vi "mainActivity_刷新界面控件.vi"(10 "控件索引2":T1, 11 "控件索引1":T2) -> (0 "错误输出":errorcluster)   [LabVIEW 2014]
uses:
  glb/glb_static.vi
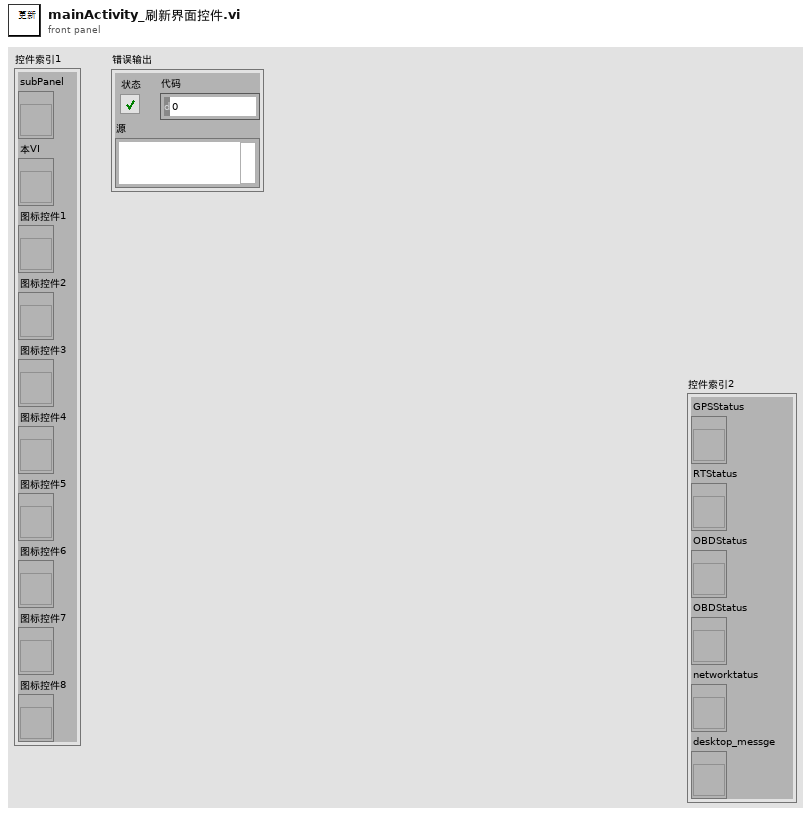
[diagram p1: front panel]
types:
  T1 = cluster{"GPSStatus":refnum<vi>, "RTStatus":refnum<vi>, "OBDStatus":refnum<vi>, "OBDStatus":refnum<vi>, "networktatus":refnum<vi>, "desktop_messge":refnum<vi>}
  T2 = cluster{"subPanel":refnum<vi>, "本VI":refnum<vi>, "图标控件1":refnum<vi>, "图标控件2":refnum<vi>, "图标控件3":refnum<vi>, "图标控件4":refnum<vi>, "图标控件5":refnum<vi>, "图标控件6":refnum<vi>, "图标控件7":refnum<vi>, "图标控件8":refnum<vi>}
  T3 = cluster{"标题":string, "相对路径":string, "类型":enum16{"服务", "活动"}, "专属队列名称":string}[]
  T4 = enum32{"Bad", "Idle", "Run top level", "Running"}
  T5 = cluster{"侧边栏数据":cluster{"来源":string, "名称":string}[], "界面刷间隔率":dbl}
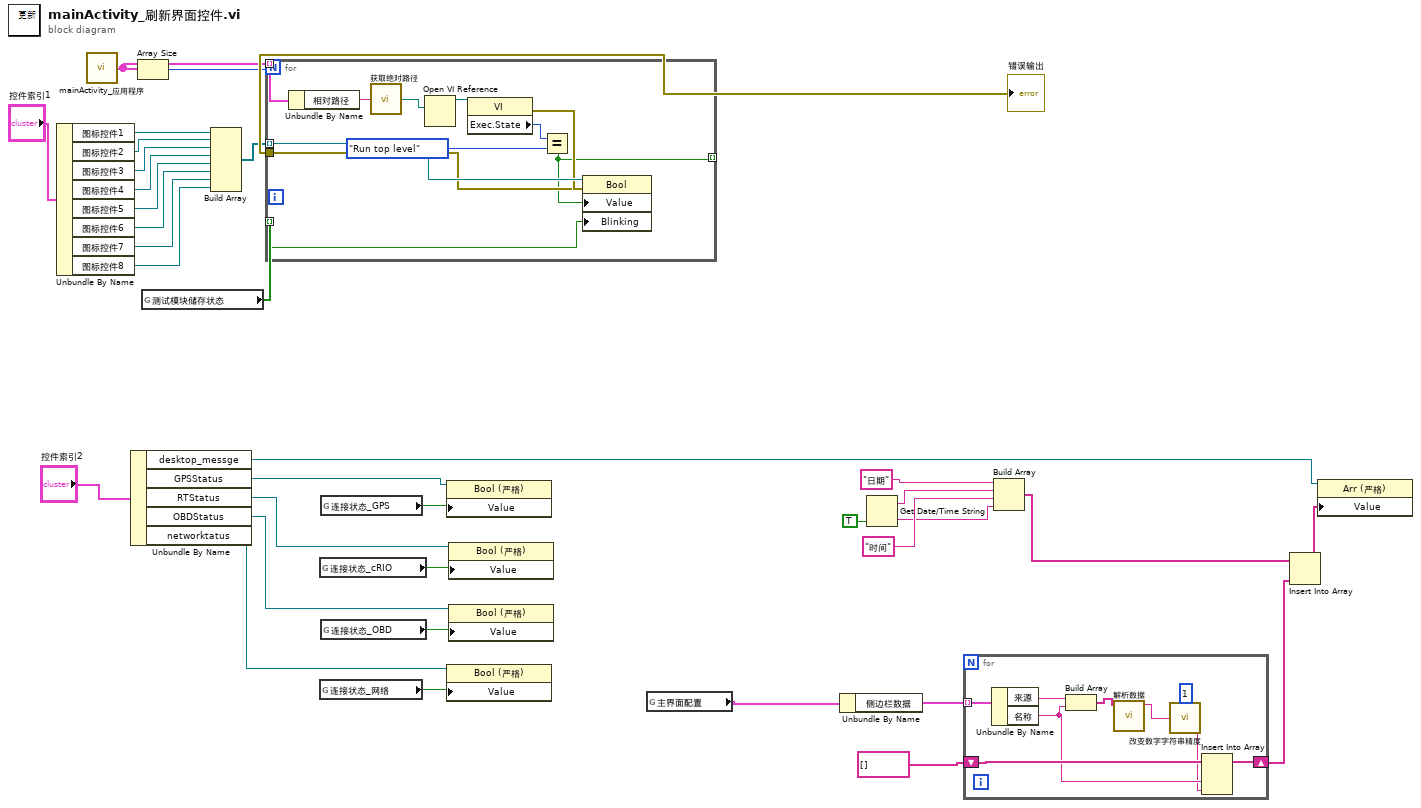
[diagram p0: block diagram]
diagram:
  n1 = Unbundle By Name("控件索引1") -> ("图标控件1"=w23:refnum<vi>, "图标控件2"=w24:refnum<vi>, "图标控件3"=w25:refnum<vi>, "图标控件4"=w26:refnum<vi>, "图标控件5"=w28:refnum<vi>, "图标控件6"=w29:refnum<vi>, "图标控件7"=w30:refnum<vi>, "图标控件8"=w31:refnum<vi>)
  n2 = call "mainActivity_应用程序.vi"() -> ("应用"=w33:T3)
  n3 = Unbundle By Name("控件索引2") -> ("desktop_messge"=w3:refnum<vi>, "GPSStatus"=w20:refnum<vi>, "RTStatus"=w15:refnum<vi>, "OBDStatus"=w14:refnum<vi>, "networktatus"=w13:refnum<vi>)
  n4 = Array Size(array=w33) -> (size(s)=w32:i32)
  n5 = global read "glb_static.vi" "测试模块储存状态"() -> (w35:bool[])
  n6 = Build Array(w23, w24, w25, w26, w28, w29, w30, w31) -> (w27:refnum<vi>[])
  n7 = for {
    N: w32 -> [_]
    tunnel: w27 -> [w43] mode=indexing
    tunnel: w33 -> [w42] mode=indexing
    tunnel: [w38] -> w34
    tunnel: w35 -> [w37] mode=indexing
    tunnel: [w36] -> _ mode=indexing
    n8 = Unbundle By Name(w42) -> ("相对路径"=w41:string)
    n9 = call "获取绝对路径.vi"("relativePath"=w41) -> ("absolutePath"=w46:path)
    n10 = Open VI Reference(vi path=w46) -> (vi reference=w45:refnum<vi>)  [unwired: 5 in, 1 out]
    n11 = property class="VI"(reference=w45) -> (error out=w39:errorcluster, "Exec.State"=w40:T4)  [unwired: 1 in, 1 out]
    n12 = Equal?(x=w40, y=T4."Run top level" ("执行:状态")) -> (x = y?=w36:bool)
    n13 = property class="Bool"(reference=w43, error in=w39, "Value"=w36, "Blinking"=w37) -> (error out=w38:errorcluster)  [unwired: 1 out]
  }
  "错误输出" <- w34
  n14 = global read "glb_static.vi" "连接状态_cRIO"() -> (w18:bool)
  n15 = global read "glb_static.vi" "连接状态_网络"() -> (w16:bool)
  n16 = global read "glb_static.vi" "连接状态_GPS"() -> (w19:bool)
  n17 = global read "glb_static.vi" "连接状态_OBD"() -> (w17:bool)
  n18 = property class="Bool (严格)"(reference=w20, "Value"=w19) -> ()  [unwired: 1 in, 2 out]
  n19 = property class="Bool (严格)"(reference=w13, "Value"=w16) -> ()  [unwired: 1 in, 2 out]
  n20 = property class="Bool (严格)"(reference=w15, "Value"=w18) -> ()  [unwired: 1 in, 2 out]
  n21 = property class="Bool (严格)"(reference=w14, "Value"=w17) -> ()  [unwired: 1 in, 2 out]
  n22 = global read "glb_static.vi" "主界面配置"() -> (w1:T5)
  n23 = Unbundle By Name(w1) -> ("侧边栏数据"=w7:cluster{"来源":string, "名称":string}[])
  n24 = Get Date/Time String(want seconds? (F)=TRUE ("需要秒？(F)")) -> (date string=w10:string, time string=w8:string)  [unwired: 2 in]
  n25 = for {
    tunnel: w7 -> [w55] mode=indexing
    shift-right: [w50] -> w4
    shift-left: string[] [] -> [w49]
    n26 = Unbundle By Name(w55) -> ("来源"=w54:string, "名称"=w48:string)
    n27 = Build Array(w54, w48) -> (w53:string[])
    n28 = call "解析数据.vi"("配置信息"=w53) -> ("输出数据"=w52:string)  [unwired: 9 in, 1 out]
    n29 = call "改变数字字符串精度.vi"("字符串"=w52, "精度位数"=u32 1) -> ("输出字符串"=w47:string)  [unwired: 1 out]
    n30 = Insert Into Array(array=w49, new element #1=w48, new element #2=w47) -> (w50:string[])  [unwired: 1 in]
  }
  n31 = Build Array("日期", w10, "时间", w8) -> (w6:string[])
  n32 = Insert Into Array(array=w6, new element=w4) -> (w2:string[])  [unwired: 1 in]
  n33 = property class="Arr (严格)"(reference=w3, "Value"=w2) -> ()  [unwired: 1 in, 2 out]
